vi "InvokeEvent.vi"(0 "Event Stream In":refnum<user-event>, 5 "Invoke?":bool=TRUE, 7 "name":string, 9 "Data":variant, 11 "error in (no error)":errorcluster) -> (4 "Event Stream Out":refnum<user-event>, 15 "error out":errorcluster)   [LabVIEW 2017]
uses:
  Types/SystemEventDataStruct.ctl
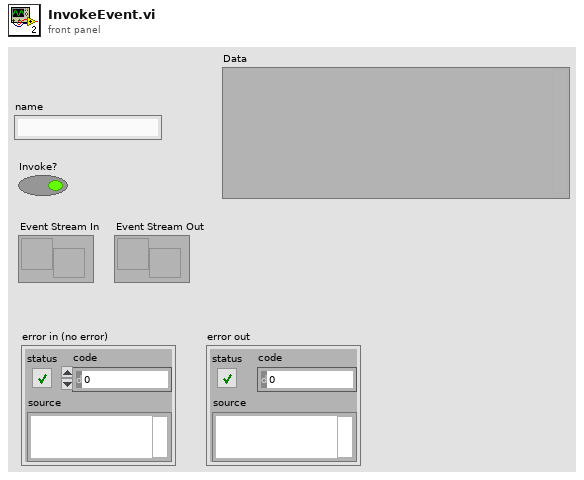
[diagram p1: front panel]
types:
  T1 = typedef "SystemEventDataStruct.ctl" = cluster{"Data":variant, "name":string}
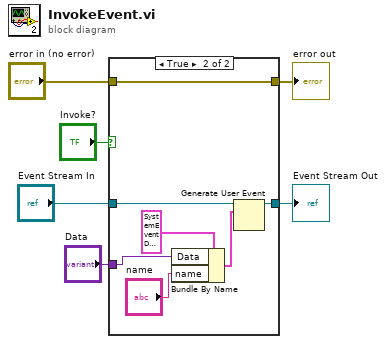
[diagram p0: block diagram]
diagram:
  n1 = case shown="True" "Invoke?" {
    tunnel: "Event Stream In" -> [w8 w12]
    tunnel: [w8 w11] -> w3
    tunnel: "error in (no error)" -> [w7 w13]
    tunnel: [w7 w13] -> w2
    tunnel: "Data" -> [_ w9]
    frame False {
    }
    frame True {
      n2 = Bundle By Name(cluster=T1 {"Data"=variant, "name"=""} ("SystemEventDataStruct"), "Data"=w9, "name"="name") -> (w10:T1)
      n3 = Generate User Event(user event=w12, event data cluster=w10) -> (user event out=w11:refnum<user-event>)  [unwired: 2 in, 1 out]
    }
  }
  "error out" <- w2
  "Event Stream Out" <- w3
